vi "BuildError.vi"(5 "Source":u16(ring)=2 items=["Caller"=2, "Caller's Caller"=3], 8 "error in (no error)":errorcluster, 10 "Source":string, 11 "Code":i32) -> (0 "error out":errorcluster)   [LabVIEW 2013, in "Advanced Plotting Toolkit.lvlib"]
uses:
  Advanced Plotting Toolkit.lvlib
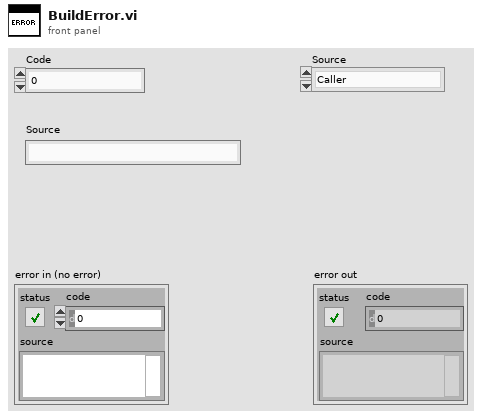
[diagram p1: front panel]
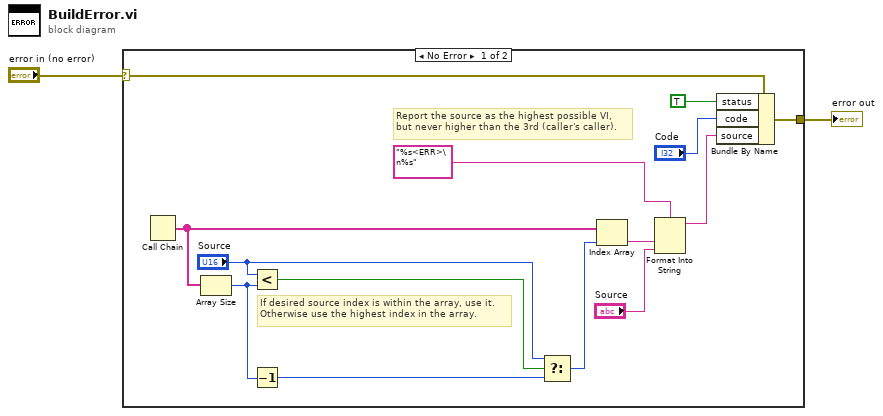
[diagram p0: block diagram]
diagram:
  n1 = case shown="No Error" "error in (no error)" {
    selector: "error in (no error)" -> [w16 w17]
    tunnel: [w10 w17] -> w1
    frame No Error {
      # "If desired source index is within the array, use it.\nOtherwise use the highest index in the array."
      # "Report the source as the highest possible VI,\nbut never higher than the 3rd (caller's caller)."
      n2 = Call Chain() -> (call chain=w12:string[])
      n3 = Array Size(array=w12) -> (size(s)=w5:i32)
      n4 = Less?(x="Source", y=w5) -> (x < y?=w6:bool)
      n5 = Decrement(x=w5) -> (x-1=w4:i32)
      n6 = Select(t="Source", s=w6, f=w4) -> (s? t:f=w7:i32)
      n7 = Index Array(array=w12, index=w7) -> (element=w8:string)
      n8 = Format Into String(format string="%s<ERR>\n%s", w8, "Source") -> (resulting string=w11:string)  [unwired: 2 in, 1 out]
      n9 = Bundle By Name(cluster=w16, "status"=TRUE, "code"="Code", "source"=w11) -> (w10:errorcluster)
    }
    frame Error {
    }
  }
  "error out" <- w1
